vi "create with existing queue.vi"(11 "identifying queue":refnum<class "identifying queue.lvclass">) -> (3 "identifying queue reporter out":refnum<class "identifying queue reporter.lvclass">)   [LabVIEW 2015, in "identifying queue reporter.lvclass"]
uses:
  identifying queue reporter.lvclass
  communicator queue/identifying queue.lvclass
  identifying queue reporter.lvclass/identifying queue reporter.ctl
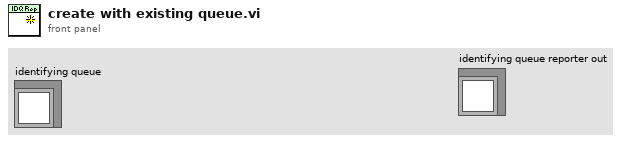
[diagram p1: front panel]
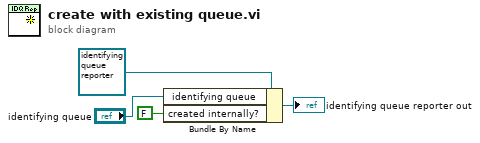
[diagram p0: block diagram]
diagram:
  n1 = Bundle By Name(cluster=refnum<class "identifying queue reporter.lvclass"> refnum ("identifying queue reporter in"), "identifying queue"="identifying queue", "created internally?"=FALSE) -> (→"identifying queue reporter out":refnum<class "identifying queue reporter.lvclass">)
